vi "Anritsu VNA Set External Trigger Mode.vi"(7 "Anritsu VNA":T2, 8 "error in (no error)":errorcluster, 10 "Ext. Trigger Mode":T1, 11 "VISA Resource Name":refnum<visa-resource-name>) -> (0 "error out":errorcluster, 2 "Previous Ext. Trigger Mode":T1, 3 "dup VISA Resource Name":refnum<visa-resource-name>)   [LabVIEW 2011]
doc: "This VI for the HP8753B Network Analyzers reads the stimulus values. Except when performing log sweeps and freq list sweeps, this VI uses the start and stop values and the number of points to calcuate the stimulus values."
uses:
  TypeDefs/Anritsu VNA External Trigger Mode.ctl
  TypeDefs/Anritsu VNA Instrument Info.ctl
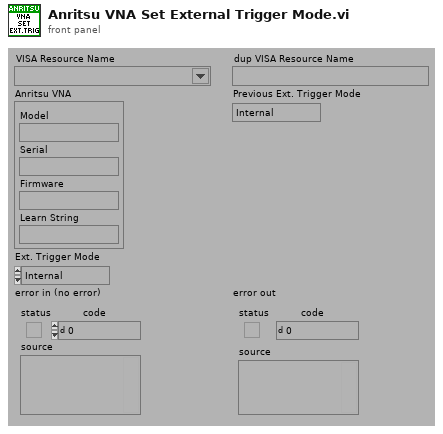
[diagram p1: front panel]
types:
  T1 = typedef "Anritsu VNA External Trigger Mode.ctl" = enum16{"Internal", "External", "Manual", "GPIB"}
  T2 = typedef "Anritsu VNA Instrument Info.ctl" = cluster{"Model":string, "Serial":string, "Firmware":string, "Learn String":string}
  T3 = typedef "Anritsu VNA Model.ctl" = enum16{"Not Supported", "37XXXX", "MS20XXX", "MS462XX", "MS464XX"}
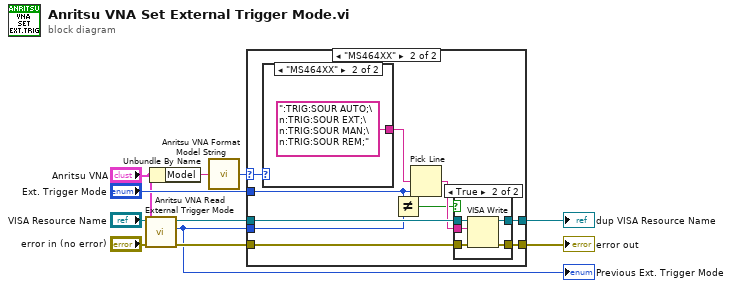
[diagram p0: block diagram]
diagram:
  n1 = call "Anritsu VNA Read External Trigger Mode.vi"("Anritsu VNA"="Anritsu VNA", "error in (no error)"="error in (no error)", "VISA Resource Name"="VISA Resource Name") -> ("error out"=w6:errorcluster, "Ext. Trigger Mode"=w4:T1, "dup VISA Resource Name"=w5:refnum<visa-resource-name>)  [unwired: 6 out]
  "Previous Ext. Trigger Mode" <- w4
  n2 = Unbundle By Name("Anritsu VNA") -> ("Model"=w3:string)
  n3 = call "Anritsu VNA Format Model String.vi"("Model"=w3) -> ("Model"=w1:T3)
  n4 = case shown="\"MS464XX\"" w1 {
    selector: w1 -> [_ w14]
    tunnel: [w13 w23] -> w11
    tunnel: [w12 w22] -> w10
    tunnel: "Ext. Trigger Mode" -> [_ w21]
    tunnel: w6 -> [w12 w20]
    tunnel: w5 -> [w13 w19]
    tunnel: w4 -> [_ w18]
    frame "Not Supported".."MS462XX" {
    }
    frame "MS464XX" {
      n5 = case shown="\"MS464XX\"" w14 {
        tunnel: [_ ":TRIG:SOUR AUTO;\n:TRIG:SOUR EXT;\n:TRIG:SOUR MAN;\n:TRIG:SOUR REM;"] -> w16
        frame "Not Supported".."MS462XX" {
        }
        frame "MS464XX" {
        }
      }
      n6 = Not Equal?(x=w21, y=w18) -> (x != y?=w15:bool)
      n7 = Pick Line(multi-line string=w16, line index=w21) -> (output string=w17:string)  [unwired: 1 out]
      n8 = case shown="True" w15 {
        tunnel: w20 -> [w25 w31]
        tunnel: w19 -> [w26 w30]
        tunnel: w17 -> [_ w29]
        tunnel: [w26 w28] -> w23
        tunnel: [w25 w27] -> w22
        frame False {
        }
        frame True {
          n9 = VISA Write(VISA resource name=w30, write buffer=w29, error in (no error)=w31) -> (VISA resource name out=w28:refnum<visa-resource-name>, error out=w27:errorcluster)  [unwired: 1 out]
        }
      }
    }
  }
  "dup VISA Resource Name" <- w11
  "error out" <- w10
